vi "test_Array DBL (Missing).vi"(8 "error in (no error)":errorcluster, 11 "TestCase in":refnum<class "Read File Tests.lvclass">) -> (0 "error out":errorcluster, 3 "TestCase out":refnum<class "Read File Tests.lvclass">)   [LabVIEW 2017, in "Read File Tests.lvclass"]
uses:
  Read File Tests.lvclass
  Read File Tests.lvclass/Read File Tests.ctl
  Read/Read Section - Array (DBL).vi
  <vilib>/addons/_JKI Toolkits/VI Tester/TestCase.llb/TestCase.lvclass
  TSC File IO.lvlib
  C:/Program Files (x86)/National Instruments/LabVIEW 2017/vi.lib/addons/_JKI Toolkits/VI Tester/TestCase.llb/TestCase.lvclass
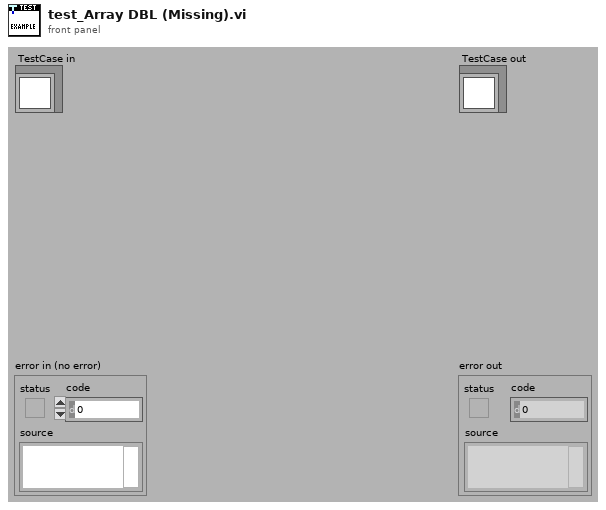
[diagram p1: front panel]
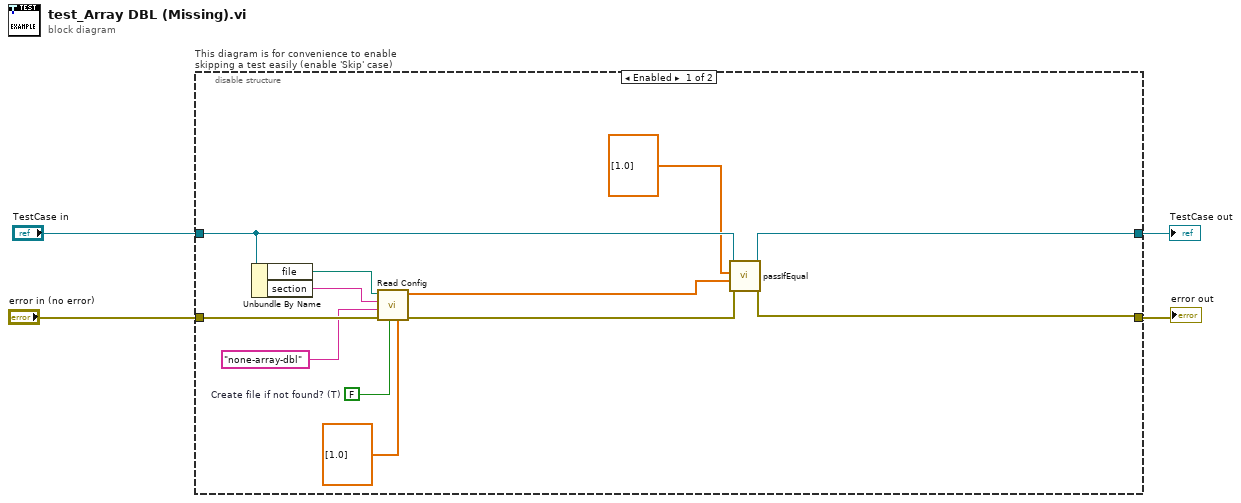
[diagram p0: block diagram]
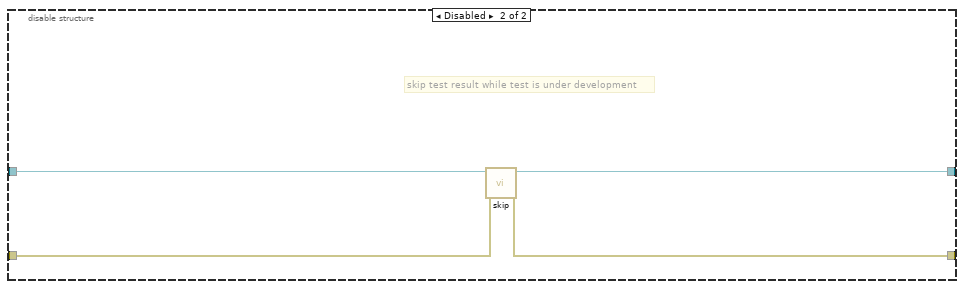
[diagram p2: hidden frame]
diagram:
  n1 = disable-structure "This diagram is for convenience to enable skipping a test easily (enable 'Skip' case)" shown="Enabled" {
    disable-tunnel: "TestCase in" -> [w14 w20]
    disable-tunnel: [w16 w18] -> w1
    disable-tunnel: [w15 w19] -> w3
    disable-tunnel: "error in (no error)" -> [w13 w17]
    frame Enabled {
      w7 = FALSE  # Create file if not found? (T)
      n2 = Unbundle By Name(w14) -> ("file"=w11:path, "section"=w10:string)
      n3 = call-poly "Read Config.vi"("Default"=dbl[] [1.0], "Create file if not found? (T)"=w7, "error in (no error)"=w13, "key"="none-array-dbl", "section"=w10, "Path"=w11) -> ("error out"=w12:errorcluster, "value"=w9:dbl[])  [unwired: 4 in]
      n4 = call-dynamic "passIfEqual.vi"("error in (no error)"=w12, "y"=w9, "x"=dbl[] [1.0], "TestCase in"=w14) -> ("error out"=w15:errorcluster, "TestCase out"=w16:refnum<class "Read File Tests.lvclass">)  [unwired: 6 in]
    }
    frame Disabled {
      # "skip test result while test is under development"
      n5 = call <vilib>:"skip.vi"("error in (no error)"=w17, "TestCase in"=w20) -> ("error out"=w19:errorcluster, "TestCase out"=w18:refnum<class "Read File Tests.lvclass">)  [unwired: 8 in]
    }
  }
  "error out" <- w3
  "TestCase out" <- w1
